vi "sv_Octave Band Frequencies.vi"(0 "octave band selector":i32, 1 "reference frequency range":u16(ring)=1 items=["Infrasonic", "Audio", "Ultrasonic"], 4 "bandwidth":T2(ring)=enum."1/3 octave", 5 "standard":T1) -> (2 "reference frequency [Hz]":dbl format="%.2f", 3 "bandedge frequencies [Hz]":cluster{"f low":dbl, "f high":dbl} {"f high" format="%.2f"; "f low" format="%.2f"}, 6 "bandwidth designator":dbl format="%.2f", 7 "midband frequency [Hz]":dbl format="%.2f")   [LabVIEW 2017, in "SoundVib_Octave_2014 standard.lvlib"]
doc: "Returns the midband and bandedge frequencies associated with a particular fractional-octave band based on the specified bandwidth and standard (ANSI or IEC).\nThe octave band selector specifies the fractional-octave band. A value of 0 corresponds to the reference frequency of the audio-frequency range, 1 kHz. Each successive value corresponds to the next fractional-octave band. Positive values cover the range above 1 kHz, and negative values cover the range below 1 kHz."
uses:
  <vilib>/addons/Sound and Vibration/svt_Octave/SoundVib_Octave_2014 standard.lvlib
  <vilib>/addons/_NISVFA/_Shared subVIs/Controls/svc_Octave Standard.ctl
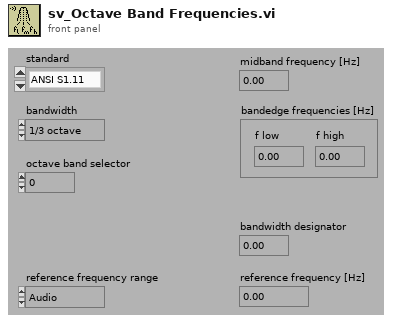
[diagram p1: front panel]
types:
  T1 = typedef "svc_Octave Standard.ctl" = enum16{"ANSI S1.11", "IEC 61260"}
  T2 = enum16{"1 octave", "1/3 octave", "1/6 octave", "1/12 octave", "1/24 octave", "1/48 octave", "1/96 octave"}
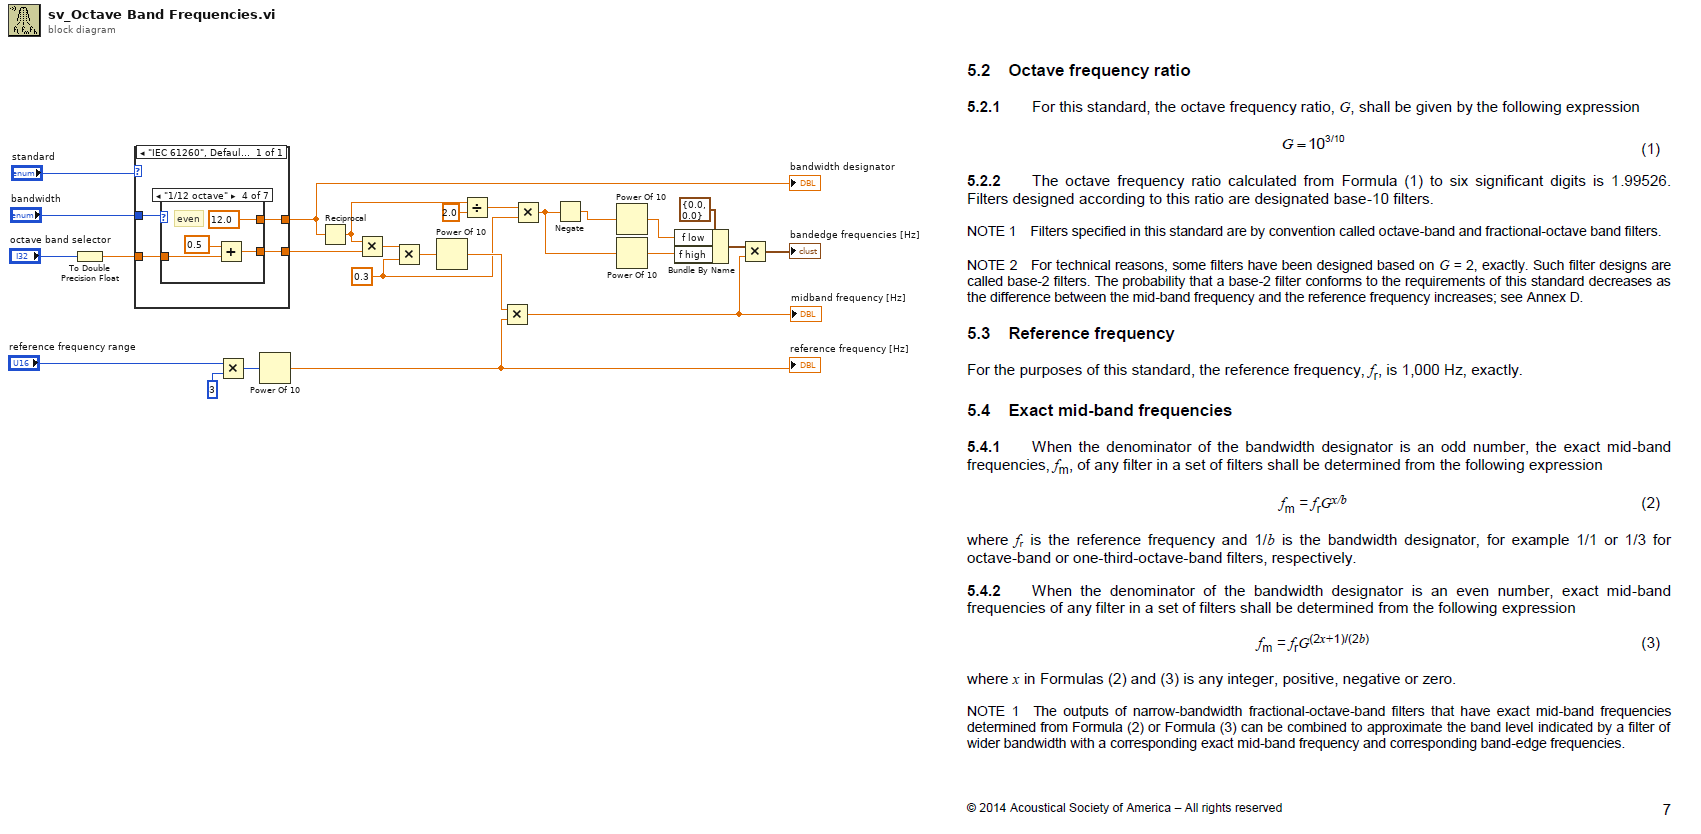
[diagram p0: block diagram]
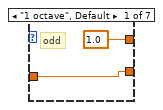
[diagram p2: hidden frame]
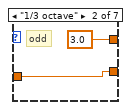
[diagram p3: hidden frame]
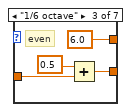
[diagram p4: hidden frame]
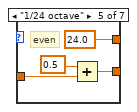
[diagram p5: hidden frame]
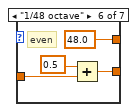
[diagram p6: hidden frame]
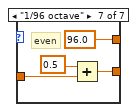
[diagram p7: hidden frame]
diagram:
  w1 = 0.3 ("y")
  n1 = To Double Precision Float(number="octave band selector") -> (double precision float=w16:dbl)
  n2 = case shown="\"IEC 61260\", Default" "standard" {
    tunnel: w16 -> [w29]
    tunnel: [w28] -> w14
    tunnel: [w27] -> w9
    tunnel: "bandwidth" -> [w26]
    frame "IEC 61260", Default {
      n3 = case shown="\"1/12 octave\"" w26 {
        tunnel: [1.0 ("x") 3.0 ("x") 6.0 ("x") 12.0 ("x") 24.0 ("x") 48.0 ("x") 96.0 ("x")] -> w27
        tunnel: w29 -> [w30 w32 w36 w39 w43 w47 w51]
        tunnel: [w30 w32 w34 w38 w42 w46 w50] -> w28
        frame "1 octave", Default {
          # "odd"
        }
        frame "1/3 octave" {
          # "odd"
        }
        frame "1/6 octave" {
          # "even"
          n4 = Add(x=0.5, y=w36) -> (x+y=w34:dbl)
        }
        frame "1/12 octave" {
          # "even"
          n5 = Add(x=0.5, y=w39) -> (x+y=w38:dbl)
        }
        frame "1/24 octave" {
          # "even"
          n6 = Add(x=0.5, y=w43) -> (x+y=w42:dbl)
        }
        frame "1/48 octave" {
          # "even"
          n7 = Add(x=0.5, y=w47) -> (x+y=w46:dbl)
        }
        frame "1/96 octave" {
          # "even"
          n8 = Add(x=0.5, y=w51) -> (x+y=w50:dbl)
        }
      }
    }
  }
  "bandwidth designator" <- w9
  n9 = Multiply(x="reference frequency range", y=u16 3) -> (x*y=w25:u16)
  n10 = Power Of 10(x=w25) -> (10^x=w6:dbl)
  "reference frequency [Hz]" <- w6
  n11 = Reciprocal(x=w9) -> (1/x=w18:dbl)
  n12 = Multiply(x=w18, y=w14) -> (x*y=w13:dbl)
  n13 = Multiply(x=w13, y=w1) -> (x*y=w12:dbl)
  n14 = Power Of 10(x=w12) -> (10^x=w17:dbl)
  n15 = Divide(x=w18, y=2.0) -> (x/y=w15:dbl)
  n16 = Multiply(x=w17, y=w6) -> (x*y=w7:dbl)
  "midband frequency [Hz]" <- w7
  n17 = Multiply(x=w15, y=w1) -> (x*y=w10:dbl)
  n18 = Negate(x=w10) -> (-x=w11:dbl)
  n19 = Power Of 10(x=w11) -> (10^x=w22:dbl)
  n20 = Power Of 10(x=w10) -> (10^x=w21:dbl)
  n21 = Bundle By Name(cluster=cluster{"f low":dbl, "f high":dbl} {"f low"=0.0, "f high"=0.0} ("bandedge frequencies [Hz] 2"), "f low"=w22, "f high"=w21) -> (w20:cluster{"f low":dbl, "f high":dbl})
  n22 = Multiply(x=w20, y=w7) -> (x*y=→"bandedge frequencies [Hz]":cluster{"f low":dbl, "f high":dbl})
